vi "Range Changer.vi"(11 "POV":i16) -> (3 "RPM":dbl format="%#_13g")   [LabVIEW 2016]
panel:
  in  "POV L RPM":dbl format="%#_13g"
  in  "POV B RPM":dbl format="%#_13g"
  in  "POV R RPM":dbl format="%#_13g"
  in  "POV F RPM":dbl format="%#_13g"
  in  "POV Left":i32=103
  in  "POV Back":i32
  in  "POV Right":i32=-43
  in  "POV Forward":i32=10
  in  "Starting Position":i32
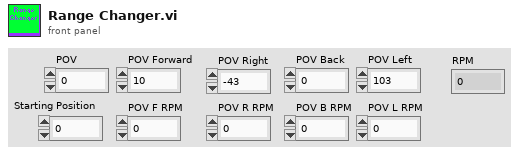
[diagram p1: front panel]
types:
  T1 = typedef "WPI_ServoDeviceRef.ctl" = cluster{"DeviceStatus":errorcluster, "PWM Channel":T2, "DeadBand":T3}
  T2 = typedef "FPGA_DIOPWMChannel.ctl" = enum8{"PWM 0", "PWM 1", "PWM 2", "PWM 3", "PWM 4", "PWM 5", "PWM 6", "PWM 7", "PWM 8", "PWM 9", "PWM MXP 0", "PWM MXP 1", "PWM MXP 2", "PWM MXP 3", "PWM MXP 4", "PWM MXP 5", "PWM MXP 6", "PWM MXP 7", "PWM MXP 8", "PWM MXP 9", "Invalid"}
  T3 = typedef "WPI_PWMDeadband.ctl" = cluster{"Name":string, "maxPositivePwm":i32, "minPositivePwm":i32, "centerPwm":i32, "maxNegativePwm":i32, "minNegativePwm":i32, "angularRange":u16}
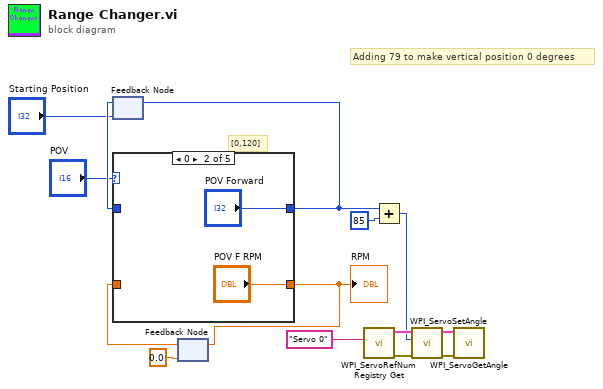
[diagram p0: block diagram]
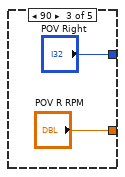
[diagram p3: hidden frame]
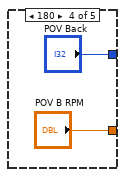
[diagram p4: hidden frame]
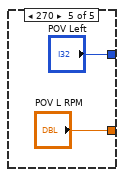
[diagram p5: hidden frame]
diagram:
  # "Adding 79 to make vertical position 0 degrees"
  # "[0,120]"
  n1 = feedback #1("Starting Position") -> (w12:i32)
  n2 = feedback #2(0.0 ("POV B RPM")) -> (w1:dbl)
  n3 = case shown="0" "POV" {
    tunnel: [w16 "POV Forward" "POV Right" "POV Back" "POV Left"] -> w7
    tunnel: w12 -> [w16 _ _ _ _]
    tunnel: [w15 "POV F RPM" "POV R RPM" "POV B RPM" "POV L RPM"] -> w3
    tunnel: w1 -> [w15 _ _ _ _]
    frame -1, Default {
    }
    frame 0 {
    }
    frame 90 {
    }
    frame 180 {
    }
    frame 270 {
    }
  }
  "RPM" <- w3
  n4 = feedback-in #1(w7) -> ()
  n5 = feedback-in #2(w3) -> ()
  n6 = call <vilib>:"WPI_ServoRefNum Registry Get.vi"("refnum name"="Servo 0") -> ("error out"=w14:errorcluster, "ServoDeviceRef"=w13:T1)  [unwired: 9 in]
  n7 = Add(x=w7, y=85) -> (x+y=w5:i32)
  n8 = call <vilib>:"WPI_ServoSetAngle.vi"("error in (no error)"=w14, "Angle"=w5, "ServoDeviceRef"=w13) -> ("error out"=w8:errorcluster, "ServoDeviceRef"=w9:T1)  [unwired: 7 in]
  n9 = call <vilib>:"WPI_ServoGetAngle.vi"("ServoDeviceRef"=w9, "error in (no error)"=w8) -> ()  [unwired: 6 in, 3 out]
